vi "ADC_Config.vi"(0 "GPIB Address":T3=8, 2 "Trigger Spec":T2={"level %(1.00)"=1.0, "slope"=enum."Rising", "Source"=enum."Free running..", "pretrigger scans (0)"=0} {"level %(1.00)" min=-100 max=100 step=1}, 5 "Ch & spans":T1[](array[typedef]) {"low limit (-10V)" format="%.3f"; "high limit (10V)" format="%.3f"}, 7 "buffer size (1000 scans)":u32=1000, 9 "scan rate (1000 scans/sec)":dbl=1000.0 format="%.2f", 11 "error in (no error)":errorcluster) -> (6 "number of channels":i32, 8 "actual scan rate":dbl format="%.2f", 15 "error out":errorcluster)   [LabVIEW 2010]
doc: "This VI configures the hardware and allocates a buffer for a buffered analog input operation for a specified group of channels. \n\nBefore performing any configuration, AI Config checks to see if the input cluster error in indicates that an error has already occurred. If so, then this VI does no configuration, but passes the error information unmodified through error out. In an error condition, taskID is 0.\n\nOtherwise, this VI calls several low-level analog input VIs to set up a task for a buffered analog input acquisition. AI Config calls Analog Input Group Config for the specified device, group, and channels to create a taskID. AI Config then calls Analog Input Hardware Config to record information about the hardware configuration. The input limits input passes to Analog Input Hardware Config, which sets up the lower and upper scaled data limits for each channel; if unspecified, the input limits do not change. This VI configures the number of AMUX boards, the coupling used for each channel (that is, AC, DC, ground, or internal reference), and the input configuration (differential, referenced single-ended, or non-referenced single ended). You can use the low-level Analog Input Hardware Config VI instead if you prefer to specify the input signal range in terms of signal range, polarity, and gain.\n\nAI Config configures the buffer for the acquisition by calling Analog Input Buffer Config. Analog Input Buffer Config allocates memory for the specified number of buffers (the default value is one), where each buffer contains buffer size number of scans.\n\nInput values:\n\n(i32) device: the number of the plug-in data acquisition board. You must specify device. \n\n([string]) channels: specifies the set of analog input channels for a group and task. You cannot assign a channel to more than one group. The default input is channel 0. See the description of the Analog Input Group Config VI for a detailed description of this parameter and the valid syntax for the channel strings.\n\n(i32) buffer size: the number of scans you want each buffer to hold. The default input is 1,000 scans.\n\n(i32) group: the number, from 0 to 15, that you assign to the specified set of channels. The default input and setting for group is 0. If you only have one acquisition for this device, the common case, you can leave this input unwired and use group 0.\n\n([cluster]) input limits: an array of clusters, of which each array element specifies the range limits for the channel(s) in the corresponding element of the channels array. If there are fewer elements in this array than in the channels array, the VI uses the last element for the rest of the channels. The default input is an empty array, which means the input limits do not change from their default settings. Each cluster contains the following parameters: \n\n (sgl) high limit: specifies the maximum scaled data the\n device measures at a particular channel.\n\n (sgl) low limit: specifies the minimum scaled data the\n device measures at a particular channel.\n\n([cluster]) coupling & input config: an array of clusters, of which each array element specifies the coupling and input configuration for the channel(s) in the corresponding element of the channels array. If there are fewer elements in this array than the number of channels, the VI uses the last element for the rest of the channels. The default input is an empty array, which means the parameters do not change from their default settings. Each cluster contains the following parameters: \n\n (u16) coupling: \n 0: Do not change the coupling setting. \n 1: DC. \n 2: AC. \n 3: Ground. \n 4: Internal reference. \n\n (u16) input config: \n 0: Do not change the input config setting. \n 1: Differential. \n 2: Referenced single-ended. \n 3: Nonreferenced single-ended. \n\n(sgl) Interchannel delay in seconds is the interval of time between two channels being sampled in your channel list.\n\n\n(i32) number of buffers: the number of buffers the VI allocates. The default input is 1 and you need to change it only for multi-buffered acquisition.\n\n(i32) number of AMUX: the number of AMUX-64T boards attached, either 0, 1, 2, or 4.\n\n(cluster) error in: a cluster describing any error conditions prior to this VI's execution. The default input of this cluster is no error. AI Config is often the first subVI in your diagram, and you may not need to wire this input. If an error has already occurred, this VI does not do the input configuration, it just passes the values of taskID in and error in to taskID out and error out. The error in cluster contains the following parameters: \n\n (bool) status: TRUE if an error has occurred.\n If status is TRUE, this VI does not do the\n input configuration.\n\n (i32) code: the error code associated with an error.\n A value of 0 means no error, a negative value is an error,\n and a positive value is a warning.\n\n (string) source: an indication of where an \n error occurred, usually the name of the VI.\n\nOutput Values:\n\n(u32) taskID: uniquely identifies the device, group, and I/O operation. Use this value as taskID in to refer to this group's operation in subsequent VIs.\n\n(i32) number of channels: the total number of channels that belong to the group, including any AMUX or SCXI channels.\n\n(cluster) error out: a cluster containing error information. If error in indicated an error, error out contains the same error information. Otherwise, it describes the error status of this VI. Use the General Error Handler utility VI to check the error at the end of your diagram. The error out cluster contains the following parameters: \n\n (bool) status: TRUE if an error has occurred.\n\n (i32) code: the error code associated with an error.\n A value of 0 means no error, a negative value is an error,\n and a positive value is a warning.\n\n (string) source: an indication of where an \n error occurred, usually the name of the VI."
uses:
  ADC_GPIB_address.ctl
  Controls/Ch_and_Spans.ctl
  Globals/Meas_global.vi
panel:
  out "SETUP STRING":string
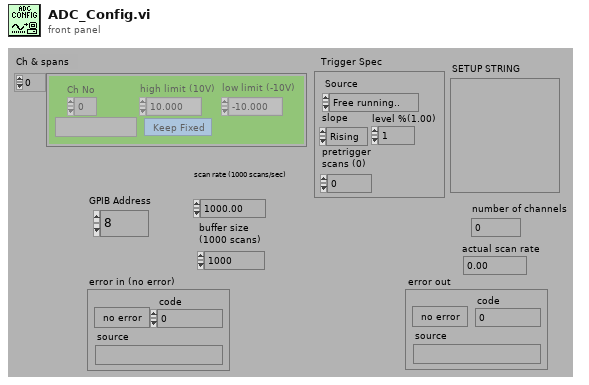
[diagram p1: front panel]
types:
  T1 = typedef "Ch_and_Spans.ctl" = cluster{"high limit (10V)":sgl, "low limit (-10V)":sgl, "Ch No":i16, "Var name":string, "Use Latest Calib":bool}
  T2 = cluster{"level %(1.00)":sgl, "slope":enum16{"Rising", "Falling"}, "Source":enum16{"Free running..", "GPIB GET", "External TTL", "First Channel", "One shot on TALK", "On shot on GET", "One shot TTL"}, "pretrigger scans (0)":u32}
  T3 = typedef "ADC_GPIB_address.ctl" = u8
  T4 = enum16{"Free running..", "GPIB GET", "External TTL", "First Channel", "One shot on TALK", "On shot on GET", "One shot TTL"}
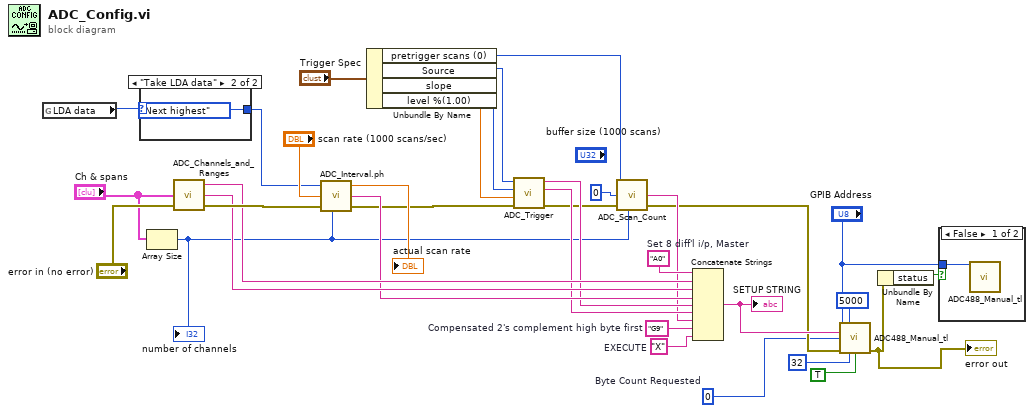
[diagram p0: block diagram]
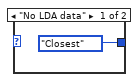
[diagram p3: hidden frame]
diagram:
  w7 = 0  # Byte Count Requested
  w15 = "X"  # EXECUTE
  w16 = "G9"  # Compensated 2's complement high byte first
  w28 = "A0"  # Set 8 diff'l i/p, Master
  n1 = global read "Meas_global.vi" "LDA data"() -> (w6:enum16{"No LDA data", "Take LDA data"})
  n2 = case shown="\"Take LDA data\"" w6 {
    tunnel: [enum16{"Closest", "Next highest"}."Closest" ("Frequency selection") enum16{"Closest", "Next highest"}."Next highest" ("Frequency selection")] -> w5
    frame "No LDA data" {
    }
    frame "Take LDA data" {
    }
  }
  n3 = Array Size(array="Ch & spans") -> (size(s)=w13:i32)
  "number of channels" <- w13
  n4 = call "ADC_Channels_and_Ranges.vi"("Ch & spans"="Ch & spans", "error in (no error)"="error in (no error)") -> ("Channel list"=w31:string, "Range list"=w30:string, "error out"=w33:errorcluster)  [unwired: 1 in, 4 out]
  n5 = call "ADC_Interval.ph.vi"("Frequency selection"=w5, "Sampling rate (Hz)"="scan rate (1000 scans/sec)", "error in (no error)"=w33, "number of channels"=w13) -> ("Actual Sampling Rate (Hz)"=→"actual scan rate":dbl, "Scan Interval"=w29:string, "error out"=w26:errorcluster)  [unwired: 3 out]
  n6 = Unbundle By Name("Trigger Spec") -> ("pretrigger scans (0)"=w17:u32, "Source"=w25:T4, "slope"=w24:enum16{"Rising", "Falling"}, "level %(1.00)"=w23:sgl)
  n7 = call "ADC_Trigger.vi"("error in (no error)"=w26, "level %(1.00)"=w23, "trigger slope"=w24, "Trigger Source"=w25) -> ("error out"=w18:errorcluster, "Level string"=w21:string, "Trigger string"=w22:string)  [unwired: 5 out]
  n8 = call "ADC_Scan_Count.vi"("pretrigger scans (0)"=w17, "post trigger scans (1000)"=u32 0, "error in (no error)"=w18, "number of channels"=w13) -> ("Scan count string"=w19:string, "error out"=w8:errorcluster)  [unwired: 4 out]
  n9 = Concatenate Strings(w28, w31, w30, w29, w22, w21, w19, w16, w15) -> (w10:string)
  "SETUP STRING" <- w10
  n10 = call "ADC488_Manual_tl.vi"("Clear device prior to command String"=TRUE, "Timeout in msec"=5000, "Serial Poll Byte"=32, "GPIB Address"="GPIB Address", "Command String"=w10, "Byte Count Requested"=w7, "error in (no error)"=w8) -> ("error out"=w3:errorcluster)  [unwired: 1 in, 7 out]
  "error out" <- w3
  n11 = Unbundle By Name(w3) -> ("status"=w2:bool)
  n12 = case shown="False" w2 {
    tunnel: "GPIB Address" -> [w37 _]
    frame False {
      n13 = call "ADC488_Manual_tl.vi"("GPIB Address"=w37) -> ()  [unwired: 7 in, 8 out]
    }
    frame True {
    }
  }
